vi "Parse Data Logger Record.vi"(8 "error in":errorcluster, 11 "Record":string[](array[string])) -> (0 "error out":errorcluster, 1 "Raw Data":dbl[][](array[numeric]), 2 "Resampled Data":waveform(dbl), 3 "Device Name":string)   [LabVIEW 2013, in "Data Log Fetcher.lvlib"]
uses:
  Data Log Fetcher.lvlib
panel:
  out "Node":string
  # "Values for E:201VAC from 19-MAR-2015 00:00:00 to 19-MAR-2015 00:01:00 from MTA\n19-MAR-2015 00:00:00.772   1.835E-07\n1 values for E:201VAC were found from MTA"
  # "No values for E:201VAC were found in the requested time interval from node MTA."
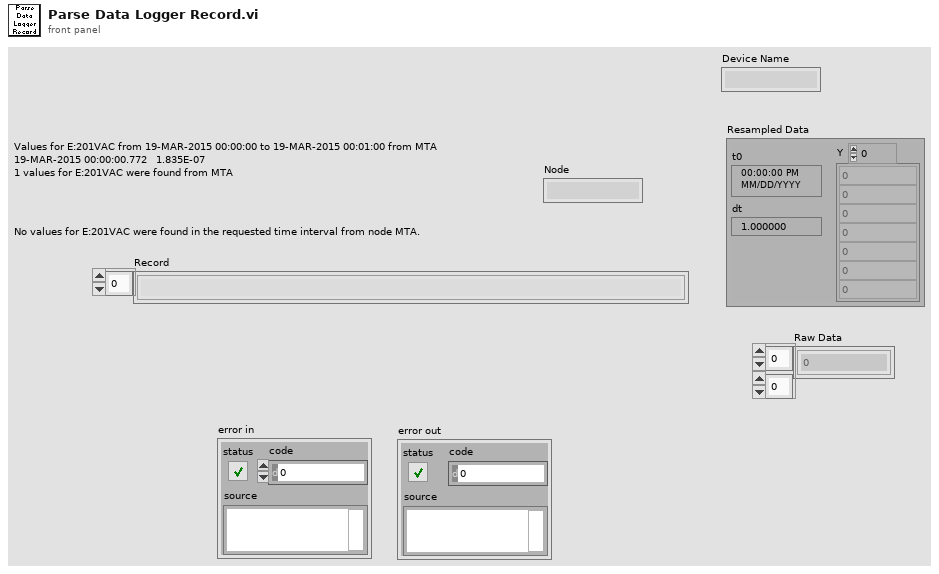
[diagram p1: front panel]
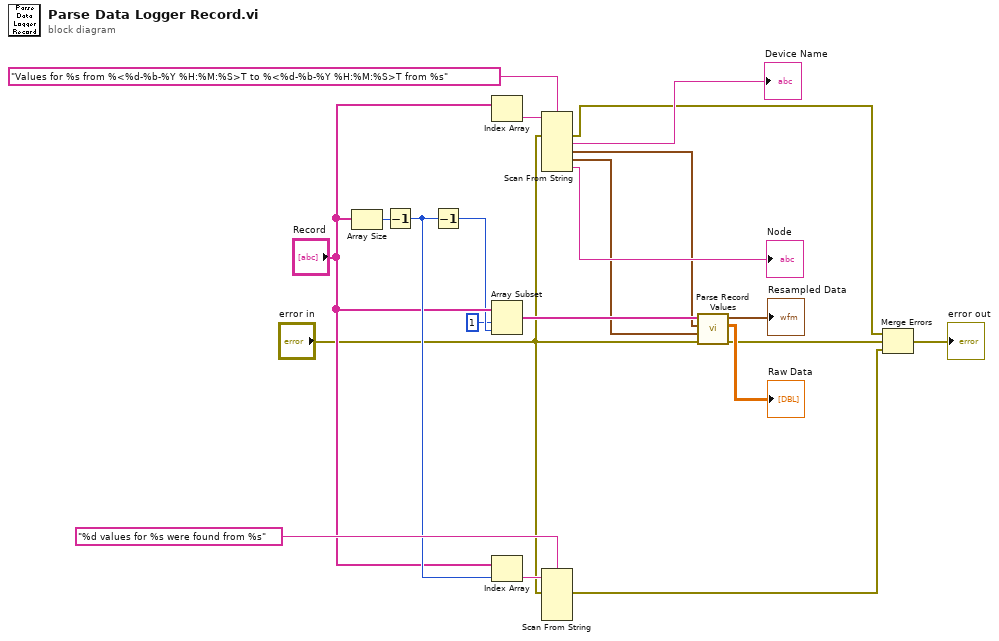
[diagram p0: block diagram]
diagram:
  n1 = Array Size(array="Record") -> (size(s)=w17:i32)
  n2 = Decrement(x=w17) -> (x-1=w14:i32)
  n3 = Decrement(x=w14) -> (x-1=w12:i32)
  n4 = Index Array(array="Record") -> (element=w20:string)  [unwired: 1 in]
  n5 = Array Subset(array="Record", index=1, length=w12) -> (w10:string[])
  n6 = Index Array(array="Record", index=w14) -> (element=w16:string)
  n7 = Scan From String(format string="Values for %s from %<%d-%b-%Y %H:%M:%S>T to %<%d-%b-%Y %H:%M:%S>T from %s", input string=w20, error in="error in") -> (error out=w4:errorcluster, output 1=→"Device Name":string, output 2=w2:timestamp, output 3=w1:timestamp, output 4=→"Node":string)  [unwired: 5 in, 2 out]
  n8 = Scan From String(format string="%d values for %s were found from %s", input string=w16, error in="error in") -> (error out=w6:errorcluster)  [unwired: 7 in, 2 out]
  n9 = call "Parse Record Values.vi"("error in"="error in", "End Time"=w1, "Start Time"=w2, "Record Values"=w10) -> ("error out"=w5:errorcluster, "Raw Data"=→"Raw Data":dbl[][], "Resampled Data"=→"Resampled Data":waveform(dbl))  [unwired: 5 in]
  n10 = Merge Errors(w4, w5, w6) -> (→"error out":errorcluster)
